vi "Get LakeShore 336 Mode.vi"(8 "error in (no error)":errorcluster, 10 "Output #":i32=1, 11 "VISA Resource Name":refnum<visa-resource-name>) -> (0 "error out":errorcluster, 1 "Control input":i32, 2 "Lake shore mode":T1, 3 "VISA Resource Name Out":refnum<visa-resource-name>, 4 "enable after power cycle":i32)   [LabVIEW 2021]
uses:
  LakeShore340/LakeShore340 Mode.ctl
  GPIB/VISA  Send Receive.vi
panel:
  out "data string out":string
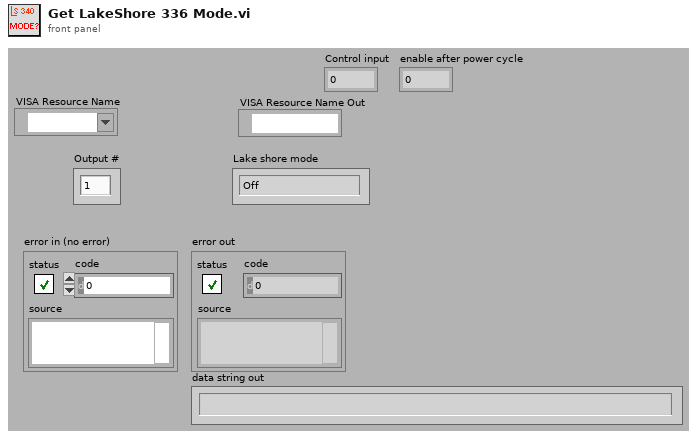
[diagram p1: front panel]
types:
  T1 = typedef "LakeShore340 Mode.ctl" = enum16{"Off", "Closed loop PID", "Zone", "Open loop", "Monitor out", "Warmup supply"}
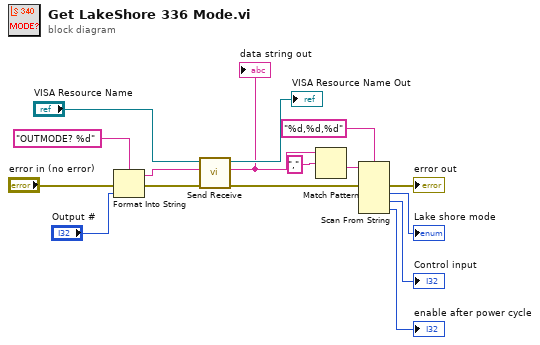
[diagram p0: block diagram]
diagram:
  n1 = Format Into String(format string="OUTMODE? %d" ("data string"), error in="error in (no error)", "Output #") -> (resulting string=w10:string, error out=w13:errorcluster)  [unwired: 1 in]
  n2 = call-poly "Send Receive.vi"("error in (no error)"=w13, "data string in"=w10, "VISA Resource Name"="VISA Resource Name") -> ("error out"=w5:errorcluster, "data string out"=w8:string, "VISA Resource Name Out"=→"VISA Resource Name Out":refnum<visa-resource-name>)  [unwired: 6 in]
  "data string out" <- w8
  n3 = Match Pattern(string=w8, regular expression=",") -> (after substring=w7:string)  [unwired: 1 in, 3 out]
  n4 = Scan From String(format string="%d,%d,%d", input string=w7, error in=w5) -> (error out=→"error out":errorcluster, output 1=→"Lake shore mode":T1, output 2=→"Control input":i32, output 3=→"enable after power cycle":i32)  [unwired: 4 in, 2 out]
